vi "start.vi"(8 "error in (no error)":errorcluster, 11 "ClockDL100201DAQmx in":refnum<class "ClockDL100201DAQmx.lvclass">) -> (0 "error out":errorcluster, 3 "ClockDL100201DAQmx out":refnum<class "ClockDL100201DAQmx.lvclass">)   [LabVIEW 2010, in "ClockDL100201DAQmx.lvclass"]
doc: "Starts the generation of the pulse trains or, if configured, arms the trigger for the operation to start"
uses:
  ClockDL100201DAQmx.lvclass
  GenericClock/GenericClock/GenericClock.lvclass
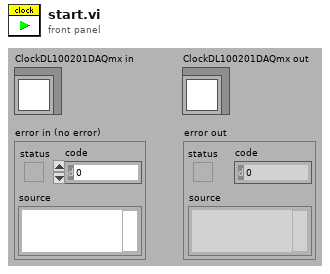
[diagram p1: front panel]
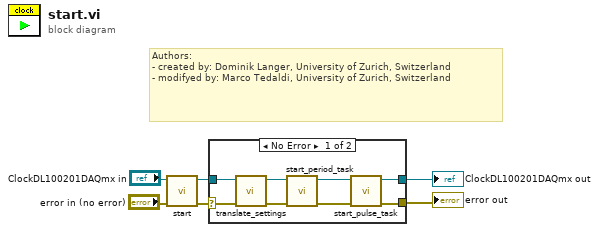
[diagram p0: block diagram]
diagram:
  # "Authors: \n- created by: Dominik Langer, University of Zurich, Switzerland\n- modifyed by: Marco Tedaldi, University of Zurich, Switzerland"
  n1 = call-parent "start.vi"("error in (no error)"="error in (no error)", "GenericClock in"="ClockDL100201DAQmx in") -> ("error out"=w4:errorcluster, "GenericClock out"=w3:refnum<class "ClockDL100201DAQmx.lvclass">)  [unwired: 8 in]
  n2 = case shown="No Error" w4 {
    selector: w4 -> [w7 w15]
    tunnel: w3 -> [w10 w16]
    tunnel: [w12 w16] -> w2
    tunnel: [w11 w15] -> w1
    frame No Error {
      n3 = call "translate_settings.vi"("error in"=w7, "GenericClock in"=w10) -> ("error out"=w8:errorcluster, "GenericClock out"=w9:refnum<class "ClockDL100201DAQmx.lvclass">)  [unwired: 6 in]
      n4 = call "start_period_task.vi"("error in"=w8, "ClockDL100201DAQmx in"=w9) -> ("error out"=w13:errorcluster, "GenericClock.lvclass out"=w14:refnum<class "ClockDL100201DAQmx.lvclass">)  [unwired: 6 in]
      n5 = call "start_pulse_task.vi"("error in"=w13, "Clock In"=w14) -> ("error out"=w11:errorcluster, "Clock Out"=w12:refnum<class "ClockDL100201DAQmx.lvclass">)  [unwired: 8 in]
    }
    frame Error {
    }
  }
  "error out" <- w1
  "ClockDL100201DAQmx out" <- w2
